vi "BRig_dataTrial_init.vi"() -> (0 "output_nCol":i32=58, 3 "output_dataTrial":u16[][](array[numeric]))   [LabVIEW 2014]
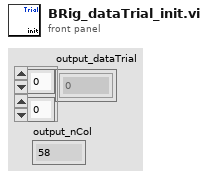
[diagram p1: front panel]
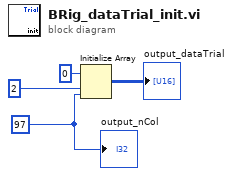
[diagram p0: block diagram]
diagram:
  w1 = 97 ("dimension size")
  n1 = Initialize Array(u16 0 ("element"), 2 ("dimension size"), w1) -> (→"output_dataTrial":u16[][])
  "output_nCol" <- w1
